vi "Main.vi"() -> ()   [LabVIEW 2017]
doc: "簡易ステートマシンデザインパターンを作成するのに、このテンプレートを使用します。各ステートはコードを実行して移行先のステートを決定します。"
uses:
  controls/State.ctl
  controls/Data.ctl
  controls/UI References.ctl
  controls/Graph Data.ctl
  controls/SQUID_data.ctl
  controls/XYZ_Data.ctl
  controls/HW Configuration.ctl
  controls/SQUID_configuration.ctl
  controls/SQUID_filter.ctl
  controls/SampleHandler_configuration.ctl
  controls/Degausser_configuration.ctl
  controls/Sequence_controll.ctl
  controls/Curret_status.ctl
  controls/wait_mode.ctl
  <vilib>/Utility/file.llb/Write Delimited Spreadsheet (string).vi
panel:
  in  "Home":bool
  out "実行中":bool
  in  "Pause":bool
  in  "Execute":bool
  in  "Save":bool
  in  "Sequence":bool
  in  "Connect":bool
  in  "Hardware setting":bool
  in  "Quit":bool
  out "文字列 2":string
  out "文字列":string
  out "RU":bool
  out "RD":bool
  out "Axis":string
  out "AF peak":u16
  out "Zero":bool
  out "Tracking":bool
  out "position (cm)":dbl
  out "Motor count":i32
  out "ARM":bool
  out "Degausser":bool
  out "Sample Handler":bool
  out "SQUID":bool
  out "数値":dbl
  out "Sequence":i32(listbox)
  out "command":i32(listbox)
  # "Status"
  # "Connection"
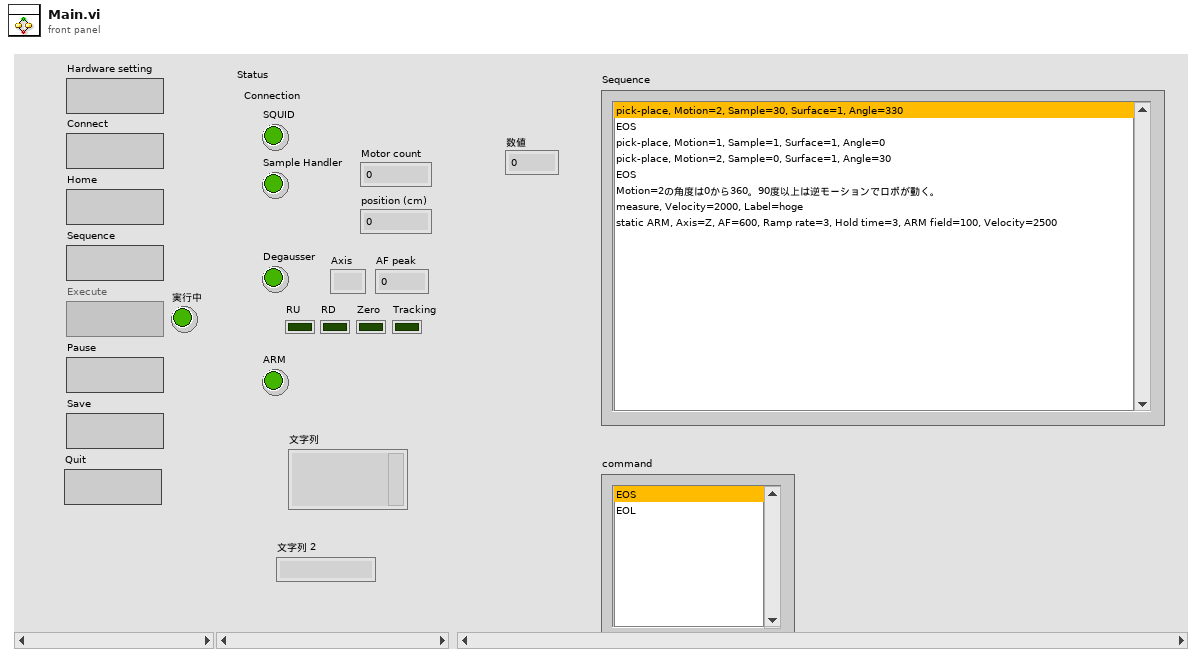
[diagram p1: front panel]
types:
  T1 = typedef "Data.ctl" = cluster{"UI ref":T2, "data":T3, "User":cluster{"Hardware configuration":T6}, "シーケンス制御":T11, "Current status":T12, "Sample offset":u16[]}
  T2 = typedef "UI References.ctl" = cluster{"Hardware setting":refnum<vi>, "Execute":refnum<vi>, "Sequence":refnum<vi>, "Pause":refnum<vi>, "Save":refnum<vi>, "Quit":refnum<vi>, "Connect":refnum<vi>}
  T3 = typedef "Graph Data.ctl" = cluster{"Label":string[], "Background":T4[], "Sample":T4[]}
  T4 = typedef "SQUID_data.ctl" = cluster{"reading":T5, "count":T5, "magnetization":T5}
  T5 = typedef "XYZ_Data.ctl" = cluster{"X":dbl, "Y":dbl, "Z":dbl}
  T6 = typedef "HW Configuration.ctl" = cluster{"SQUID":T7, "Sample Handler":T9, "Degausser":T10, "ARM Unit":cluster{"port":refnum<visa-resource-name>}, "IRM Unit（未実装）":cluster{"port":refnum<visa-resource-name>}, "Robot":cluster{"port":refnum<visa-resource-name>}}
  T7 = typedef "SQUID_configuration.ctl" = cluster{"port":refnum<visa-resource-name>, "Flux constant":T5, "X":T8, "Y":T8, "Z":T8}
  T8 = typedef "SQUID_filter.ctl" = u16
  T9 = typedef "SampleHandler_configuration.ctl" = cluster{"port":refnum<visa-resource-name>, "BG 1":i32, "BG 2":i32, "Sensor":i32, "AF 1":i32, "AF 2":i32, "AF coil":i32, "Home (absolute)":i32, "Home (relative to limit switch)":i32, "robot":i32}
  T10 = typedef "Degausser_configuration.ctl" = cluster{"port":refnum<visa-resource-name>, "Tracking timeout (sec)":i16, "Communication Delays":i16}
  T11 = typedef "Sequence_controll.ctl" = cluster{"実行中のシーケンス番号":u16, "実行中のコマンド番号":u16, "シーケンス配列":string[], "コマンド配列":string[]}
  T12 = typedef "Curret_status.ctl" = cluster{"Motor count":i32, "Degausser status":string, "Degausser axis":string, "wait mode":T13}
  T13 = typedef "wait_mode.ctl" = enum16{"Idle", "Executing", "Moving", "Homing", "Zeroing", "Ramping", "Robot", "Pause"}
  T14 = typedef "State.ctl" = enum16{"Initialize", "Update UI", "Wait for Event", "Hardware setting", "Connect", "Wait while executing", "Wait moving", "Wait homing", "Wait zero", "Wait tracking", "Wait robot", "Update command", "Exit", "Error"}
  T15 = typedef "HW_selection.ctl" = enum16{"Sample Handler", "SQUID", "Degausser", "ARM", "IRM", "Robot", "System", "Unknown"}
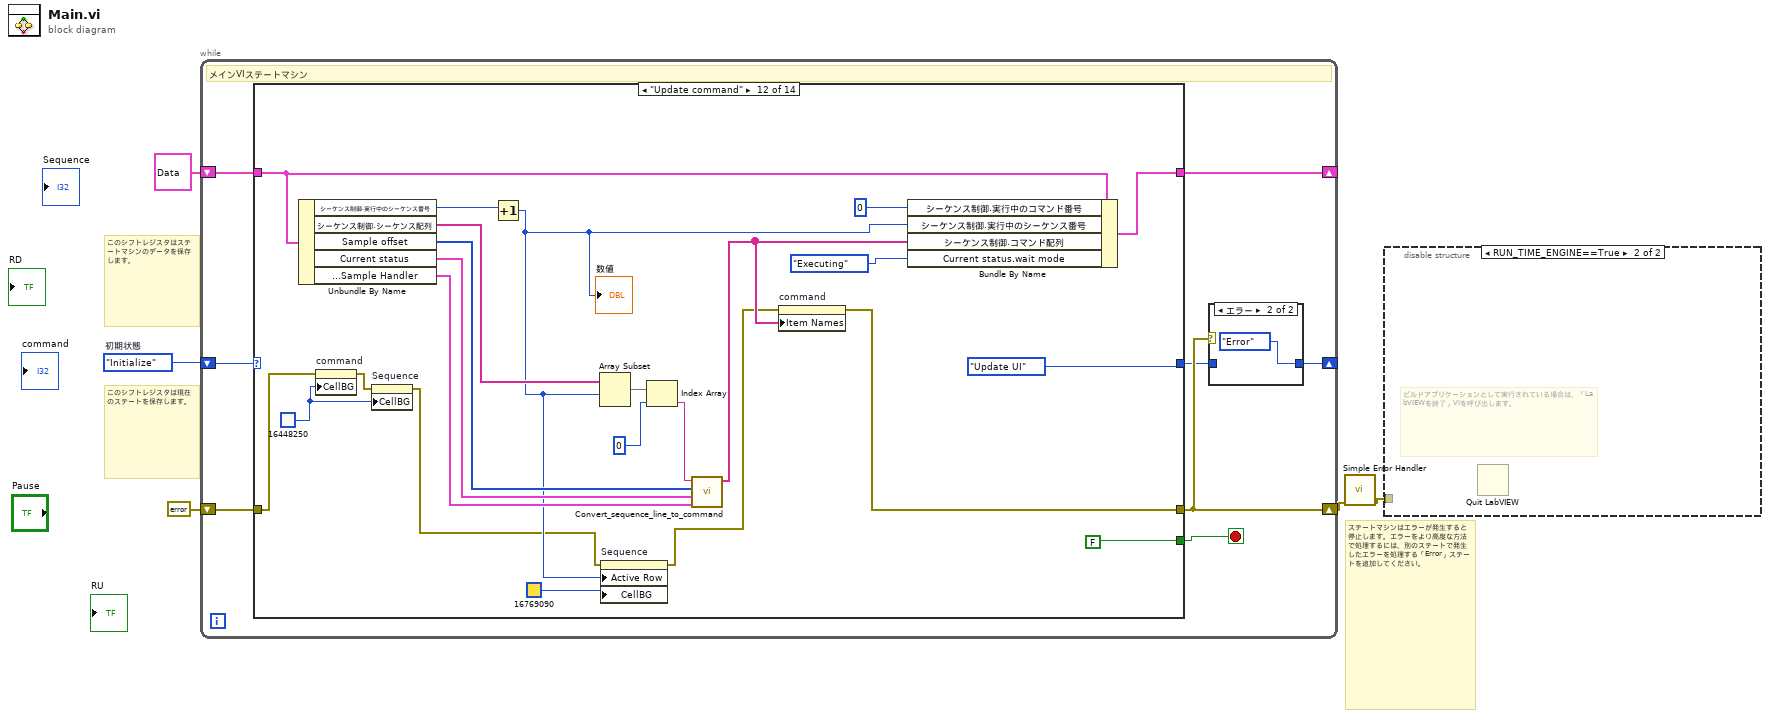
[diagram p0: block diagram]
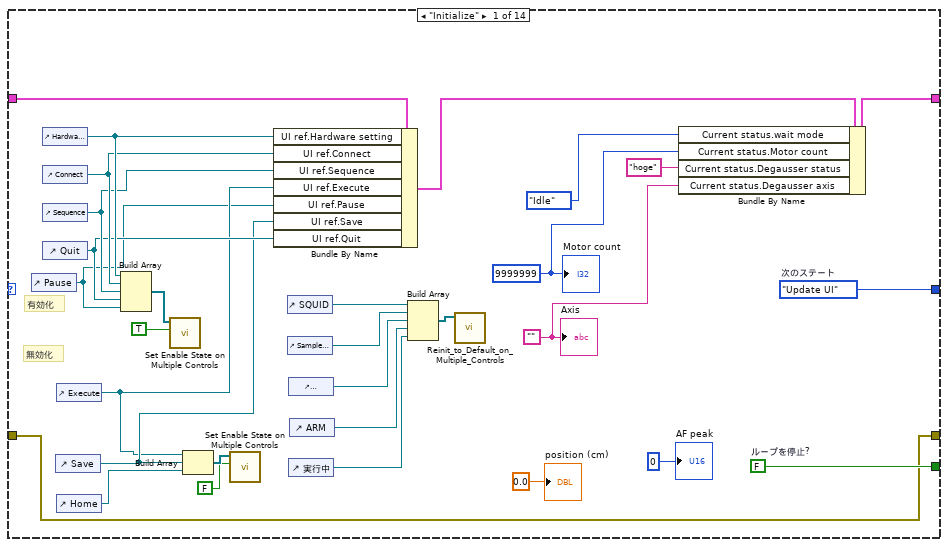
[diagram p4: hidden frame]
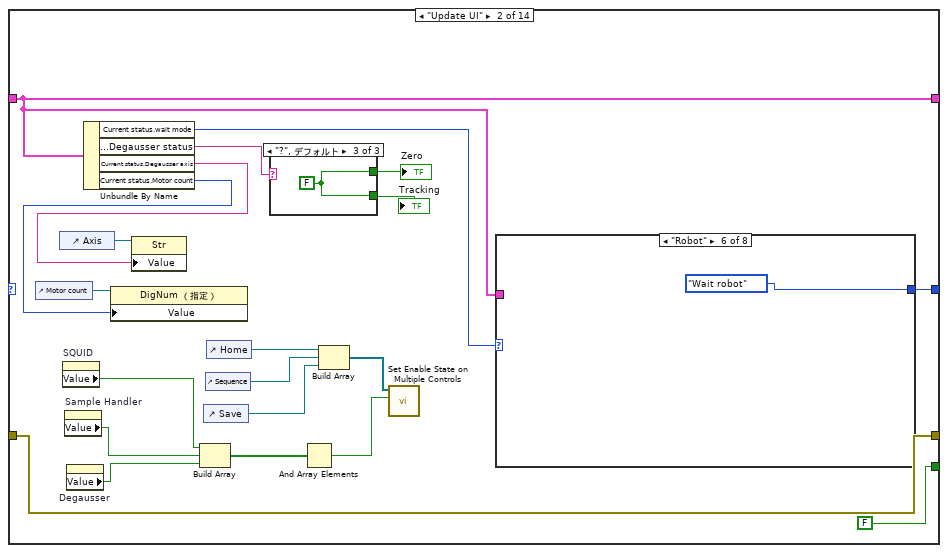
[diagram p5: hidden frame]
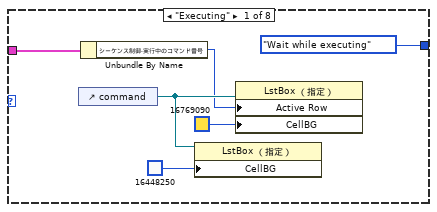
[diagram p6: hidden frame]
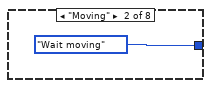
[diagram p7: hidden frame]
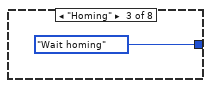
[diagram p8: hidden frame]
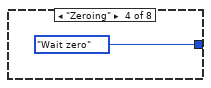
[diagram p9: hidden frame]
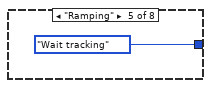
[diagram p10: hidden frame]
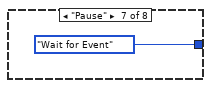
[diagram p11: hidden frame]
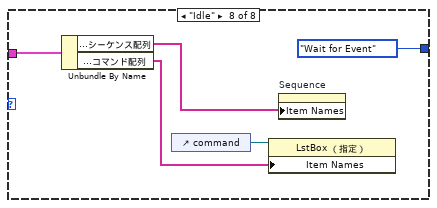
[diagram p12: hidden frame]
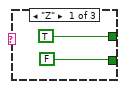
[diagram p13: hidden frame]
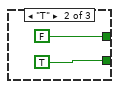
[diagram p14: hidden frame]
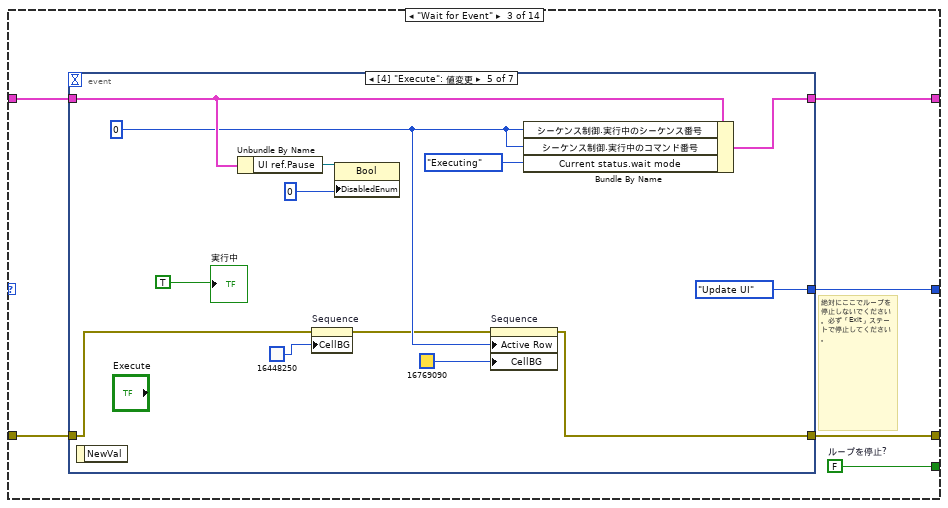
[diagram p15: hidden frame]
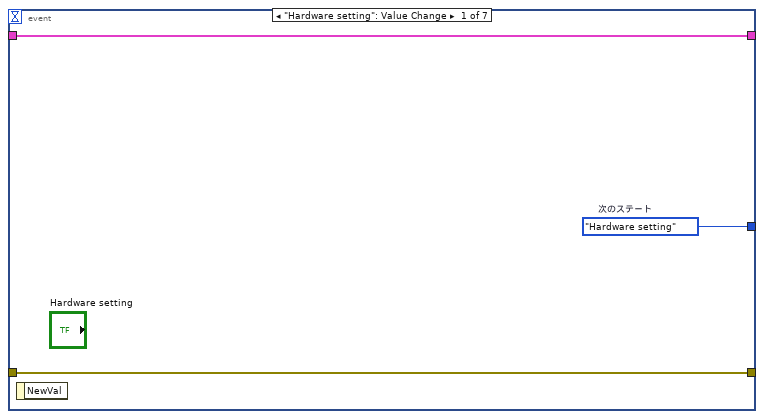
[diagram p16: hidden frame]
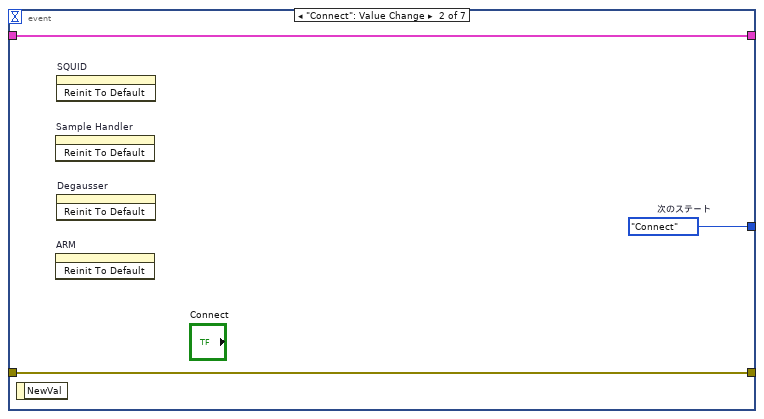
[diagram p17: hidden frame]
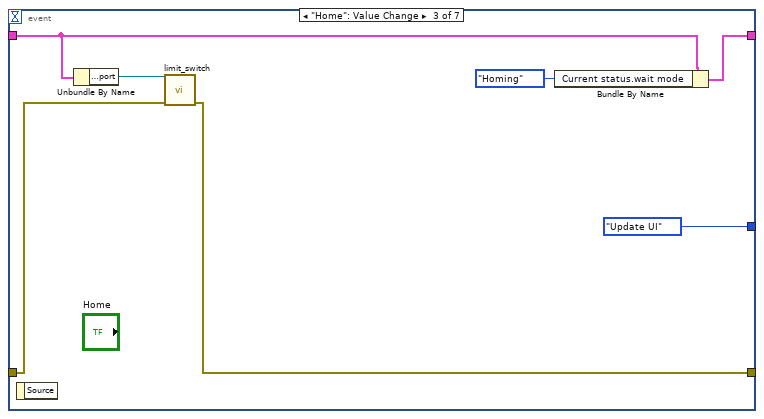
[diagram p18: hidden frame]
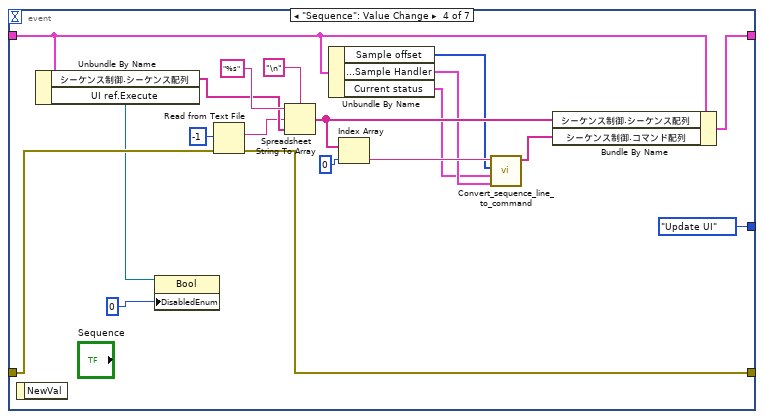
[diagram p19: hidden frame]
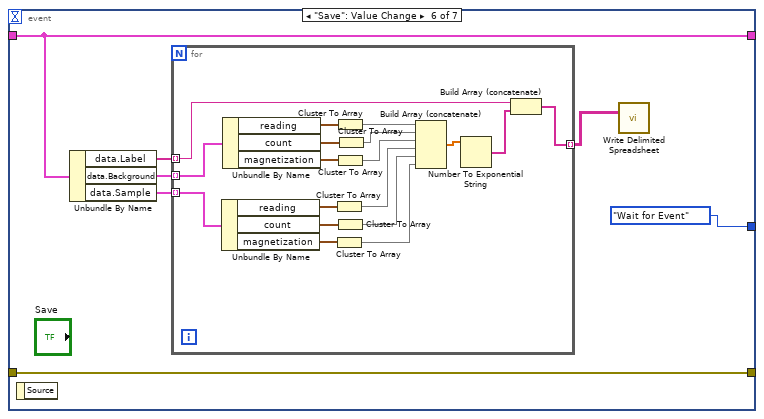
[diagram p20: hidden frame]
diagram:
  w5 = State."Initialize"  # 初期状態
  # "ステートマシンはエラーが発生すると停止します。エラーをより高度な方法で処理するには、別のステートで発生したエラーを処理する「Error」ステートを追加してください。"
  # "このシフトレジスタはステートマシンのデータを保存します。"
  # "このシフトレジスタは現在のステートを保存します。"
  n1 = while {
    shift-right: [w7] -> _
    shift-left: w5 -> [w13]
    shift-right: [w12] -> _
    shift-left: T1 {"UI ref"={"Hardware setting"=refnum, "Execute"=refnum, "Sequence"=refnum, "Pause"=refnum, "Save"=refnum, "Quit"=refnum, "Connect"=refnum}, "data"={"Label"=[], "Background"=[], "Sample"=[]}, "User"={"Hardware configuration"={"SQUID"={"port"="", "Flux constant"={"X"=0.0, "Y"=0.0, "Z"=0.0}, "X"=0, "Y"=0, "Z"=0}, "Sample Handler"={"port"="", "BG 1"=0, "BG 2"=0, "Sensor"=0, "AF 1"=0, "AF 2"=0, "AF coil"=0, "Home (absolute)"=0, "Home (relative to limit switch)"=0, "robot"=40750}, "Degausser"={"port"="", "Tracking timeout (sec)"=0, "Communication Delays"=0}, "ARM Unit"={"port"=""}, "IRM Unit（未実装）"={"port"=""}, "Robot"={"port"=""}}}, "シーケンス制御"={"実行中のシーケンス番号"=0, "実行中のコマンド番号"=0, "シーケンス配列"=[], "コマンド配列"=[]}, "Current status"={"Motor count"=0, "Degausser status"="", "Degausser axis"="", "wait mode"=enum."Idle"}, "Sample offset"=[37618]} ("Data") -> [w10]
    shift-right: [w9] -> w2
    shift-left: errorcluster {"status"=FALSE, "code"=0, "source"=""} ("error constant") -> [w11]
    stop <- w6 stop-if-true
    # "メインVIステートマシン"
    n2 = case shown="\"Update command\"" w13 {
      tunnel: [w45 w66 w94 w173 w199 w208 w406 w453 w492 w516 State."Wait tracking" ("ステート") State."Update UI" ("ステート") w588 State."Exit" ("ステート")] -> w8
      tunnel: [w44 FALSE w93 FALSE ("Stop Loop?") FALSE ("Stop Loop?") w214 FALSE FALSE FALSE FALSE FALSE FALSE w587 FALSE] -> w6
      tunnel: w10 -> [w34 w47 w92 w169 w197 w213 w403 w450 w495 w519 w545 w553 w578 w592]
      tunnel: [w23 w47 w91 w168 w196 w212 w402 w449 w494 w518 w545 w552 w578 w592] -> w12
      tunnel: w11 -> [w33 w56 w90 w171 w193 w211 w401 w448 w498 w521 w544 w563 w579 w591]
      tunnel: [w33 w56 w89 w171 w175 w209 w400 w447 w497 w515 w544 w557 w569 w591] -> w9
      frame "Initialize" {
        w19 = ""
        w21 = 9999999
        w44 = FALSE  # ループを停止?
        w45 = State."Update UI"  # 次のステート
        # "無効化"
        # "有効化"
        # "Initialize ― アプリケーションを初期化します。"
        n3 = control-ref of="Pause"() -> (w16:refnum<vi>)
        n4 = control-ref of="Hardware setting"() -> (w32:refnum<vi>)
        n5 = control-ref of="Connect"() -> (w31:refnum<vi>)
        n6 = control-ref of="Sequence"() -> (w30:refnum<vi>)
        n7 = control-ref of="Quit"() -> (w29:refnum<vi>)
        n8 = control-ref of="Save"() -> (w28:refnum<vi>)
        n9 = control-ref of="Execute"() -> (w17:refnum<vi>)
        n10 = control-ref of="Home"() -> (w18:refnum<vi>)
        n11 = Build Array(w32, w31, w30, w29, w16) -> (w43:refnum<vi>[])
        n12 = call "Set Enable State on Multiple Controls.vi"("有効?"=TRUE, "制御器"=w43) -> ()  [unwired: 10 in]
        n13 = Build Array(w17, w28, w18) -> (w41:refnum<vi>[])
        n14 = call "Set Enable State on Multiple Controls.vi"("有効?"=FALSE, "制御器"=w41) -> ()  [unwired: 10 in]
        n15 = Bundle By Name(cluster=w34, "UI ref.Hardware setting"=w32, "UI ref.Connect"=w31, "UI ref.Sequence"=w30, "UI ref.Execute"=w17, "UI ref.Pause"=w16, "UI ref.Save"=w28, "UI ref.Quit"=w29) -> (w24:T1)
        n16 = control-ref of="SQUID"() -> (w39:refnum<vi>)
        n17 = control-ref of="Sample Handler"() -> (w38:refnum<vi>)
        n18 = control-ref of="Degausser"() -> (w36:refnum<vi>)
        n19 = control-ref of="実行中"() -> (w22:refnum<vi>)
        n20 = control-ref of="ARM"() -> (w35:refnum<vi>)
        n21 = Build Array(w39, w38, w36, w35, w22) -> (w37:refnum<vi>[])
        n22 = call "Reinit_to_Default_on_Multiple_Controls.vi"("配列"=w37) -> ()  [unwired: 11 in]
        n23 = Bundle By Name(cluster=w24, "Current status.wait mode"=wait_mode."Idle" ("wait mode"), "Current status.Motor count"=w21, "Current status.Degausser status"="hoge", "Current status.Degausser axis"=w19) -> (w23:T1)
        "Motor count" <- w21
        "Axis" <- w19
        "AF peak" <- 0
        "position (cm)" <- 0.0
      }
      frame "Update UI" {
        n24 = control-ref of="Motor count"() -> (w60:refnum<vi>)
        n25 = control-ref of="Axis"() -> (w62:refnum<vi>)
        n26 = property on="SQUID" class="Bool （指定）"() -> ("Value"=w51:bool)  [unwired: 2 in, 2 out]
        n27 = property on="Sample Handler" class="Bool （指定）"() -> ("Value"=w50:bool)  [unwired: 2 in, 2 out]
        n28 = property on="Degausser" class="Bool （指定）"() -> ("Value"=w49:bool)  [unwired: 2 in, 2 out]
        n29 = Unbundle By Name(w47) -> ("Current status.wait mode"=w57:T13, "Current status.Degausser status"=w65:string, "Current status.Degausser axis"=w61:string, "Current status.Motor count"=w59:i32)
        n30 = property class="DigNum （指定）"(reference=w60, "Value"=w59) -> ()  [unwired: 1 in, 2 out]
        n31 = property class="Str"(reference=w62, "Value"=w61) -> ()  [unwired: 1 in, 2 out]
        n32 = Build Array(w51, w50, w49) -> (w48:bool[])
        n33 = control-ref of="Save"() -> (w46:refnum<vi>)
        n34 = control-ref of="Sequence"() -> (w52:refnum<vi>)
        n35 = control-ref of="Home"() -> (w53:refnum<vi>)
        n36 = case shown="\"?\", デフォルト" w65 {
          tunnel: [TRUE FALSE w88] -> w64
          tunnel: [FALSE TRUE w88] -> w63
          frame "Z" {
          }
          frame "T" {
          }
          frame "?", Default {
            w88 = FALSE
          }
        }
        "Zero" <- w64
        "Tracking" <- w63
        n37 = And Array Elements(Boolean array=w48) -> (logical AND=w54:bool)
        n38 = Build Array(w53, w52, w46) -> (w55:refnum<vi>[])
        n39 = call "Set Enable State on Multiple Controls.vi"("有効?"=w54, "制御器"=w55) -> ()  [unwired: 10 in]
        n40 = case shown="\"Robot\"" w57 {
          tunnel: [State."Wait while executing" ("ステート") State."Wait moving" ("ステート") State."Wait homing" ("ステート") State."Wait zero" ("ステート") State."Wait tracking" ("ステート") State."Wait robot" ("ステート") State."Wait for Event" ("ステート") State."Wait for Event" ("ステート")] -> w66
          tunnel: w47 -> [w68 _ _ _ _ _ _ w81]
          frame "Executing" {
            n41 = control-ref of="command"() -> (w71:refnum<vi>)
            n42 = Unbundle By Name(w68) -> ("シーケンス制御.実行中のコマンド番号"=w67:u16)
            n43 = property class="LstBox （指定）"(reference=w71, "CellBG"=u32 16448250) -> ()  [unwired: 1 in, 2 out]
            n44 = property class="LstBox （指定）"(reference=w71, "Active Row"=w67, "CellBG"=u32 16769090) -> ()  [unwired: 1 in, 2 out]
          }
          frame "Moving" {
          }
          frame "Homing" {
          }
          frame "Zeroing" {
          }
          frame "Ramping" {
          }
          frame "Robot" {
          }
          frame "Pause" {
          }
          frame "Idle" {
            n45 = Unbundle By Name(w81) -> ("シーケンス制御.シーケンス配列"=w79:string[], "シーケンス制御.コマンド配列"=w80:string[])
            n46 = control-ref of="command"() -> (w82:refnum<vi>)
            n47 = property class="LstBox （指定）"(reference=w82, "Item Names"=w80) -> ()  [unwired: 1 in, 2 out]
            n48 = property on="Sequence" class="LstBox （指定）"("Item Names"=w79) -> ()  [unwired: 2 in, 2 out]
          }
        }
      }
      frame "Wait for Event" {
        w93 = FALSE  # ループを停止?
        # "絶対にここでループを停止しないでください。必ず「Exit」ステートで停止してください。"
        # "Wait for Event - イベントストラクチャを使用し、ステートマシンの各ステートを実行するユーザインタフェースイベントの発生を監視します。"
        n49 = event shown="[4] \"Execute\": 値変更" {
          selector: _ -> [_ _ _ _ _ _ _]
          dyn-events: _ -> [_ _ _ _ _ _ _]
          timeout: _ -> [_ _ _ _ _ _ _]
          tunnel: [w97 w100 State."Update UI" ("ステート") State."Update UI" ("ステート") State."Update UI" ("ステート") State."Wait for Event" ("ステート") w167] -> w94
          tunnel: w92 -> [w95 w98 w105 w113 w136 w145 w166]
          tunnel: [w95 w98 w106 w123 w138 w145 w166] -> w91
          tunnel: w90 -> [w96 w99 w103 w126 w130 w146 w165]
          tunnel: [w96 w99 w102 w121 w127 w146 w165] -> w89
          event "Hardware setting": Value Change {
            w97 = State."Hardware setting"  # 次のステート
            n50 = event-data() -> ()  [unwired: 1 in, 1 out]
          }
          event "Connect": Value Change {
            w100 = State."Connect"  # 次のステート
            n51 = event-data() -> ()  [unwired: 1 in, 1 out]
            n52 = invoke on="Sample Handler" class="Bool （指定）" method="Reinit To Default"() -> ()  [unwired: 3 in, 3 out]
            n53 = invoke on="ARM" class="Bool （指定）" method="Reinit To Default"() -> ()  [unwired: 3 in, 3 out]
            n54 = invoke on="SQUID" class="Bool （指定）" method="Reinit To Default"() -> ()  [unwired: 3 in, 3 out]
            n55 = invoke on="Degausser" class="Bool （指定）" method="Reinit To Default"() -> ()  [unwired: 3 in, 3 out]
          }
          event "Home": Value Change {
            n56 = event-data() -> ()  [unwired: 1 in, 1 out]
            n57 = Unbundle By Name(w105) -> ("User.Hardware configuration.Sample Handler.port"=w104:refnum<visa-resource-name>)
            n58 = call "limit_switch.vi"("error in (no error)"=w103, "VISAリソース名"=w104) -> ("error out"=w102:errorcluster)  [unwired: 8 in, 1 out]
            n59 = Bundle By Name(cluster=w105, "Current status.wait mode"=wait_mode."Homing" ("wait mode")) -> (w106:T1)
          }
          event "Sequence": Value Change {
            n60 = event-data() -> ()  [unwired: 1 in, 1 out]
            n61 = Unbundle By Name(w113) -> ("シーケンス制御.シーケンス配列"=w109:string[], "UI ref.Execute"=w119:refnum<vi>)
            n62 = property class="Bool"(reference=w119, "DisabledEnum"=0) -> ()  [unwired: 1 in, 2 out]
            n63 = Read from Text File(count=-1, error in=w126) -> (text=w108:string, error out=w121:errorcluster)  [unwired: 2 in, 2 out]
            n64 = Spreadsheet String To Array(delimiter (Tab)="\n", format string="%s", spreadsheet string=w108, array type (2D Dbl)=w109) -> (array=w117:string[])
            n65 = Unbundle By Name(w113) -> ("Sample offset"=w110:u16[], "User.Hardware configuration.Sample Handler"=w112:T9, "Current status"=w111:T12)
            n66 = Index Array(array=w117, index=0) -> (element=w115:string)
            n67 = call "Convert_sequence_line_to_command.vi"("Sample Handler Configuration"=w112, "Current status"=w111, "Sample offset"=w110, "sequence line"=w115) -> ("コマンド配列"=w114:string[])  [unwired: 7 in]
            n68 = Bundle By Name(cluster=w113, "シーケンス制御.シーケンス配列"=w117, "シーケンス制御.コマンド配列"=w114) -> (w123:T1)
          }
          event "Execute": Value Change {
            w132 = 0
            n69 = event-data() -> ()  [unwired: 1 in, 1 out]
            n70 = Unbundle By Name(w136) -> ("UI ref.Pause"=w135:refnum<vi>)
            n71 = property on="Sequence" class="LstBox （指定）"(error in=w130, "CellBG"=u32 16448250) -> (error out=w128:errorcluster)  [unwired: 1 in, 1 out]
            n72 = property class="Bool"(reference=w135, "DisabledEnum"=0) -> ()  [unwired: 1 in, 2 out]
            n73 = property on="Sequence" class="LstBox （指定）"(error in=w128, "Active Row"=w132, "CellBG"=u32 16769090) -> (error out=w127:errorcluster)  [unwired: 1 in, 1 out]
            n74 = Bundle By Name(cluster=w136, "シーケンス制御.実行中のシーケンス番号"=w132, "シーケンス制御.実行中のコマンド番号"=w132, "Current status.wait mode"=wait_mode."Executing" ("wait mode")) -> (w138:T1)
            "実行中" <- TRUE
          }
          event "Save": Value Change {
            n75 = event-data() -> ()  [unwired: 1 in, 1 out]
            n76 = Unbundle By Name(w145) -> ("data.Label"=w140:string[], "data.Background"=w141:T4[], "data.Sample"=w144:T4[])
            n77 = for {
              tunnel: w144 -> [w160] mode=indexing
              tunnel: [w161] -> w143 mode=indexing
              tunnel: w141 -> [w156] mode=indexing
              tunnel: w140 -> [w148] mode=indexing
              n78 = Unbundle By Name(w160) -> ("reading"=w164:T5, "count"=w162:T5, "magnetization"=w163:T5)
              n79 = Unbundle By Name(w156) -> ("reading"=w159:T5, "count"=w157:T5, "magnetization"=w158:T5)
              n80 = Cluster To Array(cluster=w164) -> (array=w152:dbl[])
              n81 = Cluster To Array(cluster=w163) -> (array=w150:dbl[])
              n82 = Cluster To Array(cluster=w159) -> (array=w155:dbl[])
              n83 = Cluster To Array(cluster=w158) -> (array=w153:dbl[])
              n84 = Cluster To Array(cluster=w162) -> (array=w151:dbl[])
              n85 = Cluster To Array(cluster=w157) -> (array=w154:dbl[])
              n86 = Build Array (concatenate)(w155, w154, w153, w152, w151, w150) -> (w149:dbl[])
              n87 = Number To Exponential String(number=w149) -> (E-format string=w147:string[])  [unwired: 3 in]
              n88 = Build Array (concatenate)(w148, w147) -> (w161:string[])
            }
            n89 = call-poly <vilib>:"Write Delimited Spreadsheet.vi"("2D data"=w143) -> ()  [unwired: 13 in, 2 out]
          }
          event "Quit": Value Change {
            w167 = State."Exit"  # 次のステート
            n90 = event-data() -> ()  [unwired: 1 in, 1 out]
          }
        }
      }
      frame "Hardware setting" {
        w173 = State."Wait for Event"  # 次のステート
        # "User State 1 - このステートをユーザ自身のアプリケーションの機能と置換します。"
        n91 = call "Configure_HW_dialog.vi"() -> ("output"=w170:T6)  [unwired: 11 in]
        n92 = Bundle By Name(cluster=w169, "User.Hardware configuration"=w170) -> (w168:T1)
      }
      frame "Connect" {
        w199 = State."Update UI"  # 次のステート
        # "User State 2 - このステートをユーザ自身のアプリケーションの機能と置換します。"
        n93 = Unbundle By Name(w197) -> ("User.Hardware configuration.SQUID.port"=w194:refnum<visa-resource-name>, "User.Hardware configuration.Sample Handler.port"=w192:refnum<visa-resource-name>, "User.Hardware configuration.Degausser.port"=w189:refnum<visa-resource-name>, "User.Hardware configuration.Degausser.Communication Delays"=w188:i16, "User.Hardware configuration.ARM Unit.port"=w186:refnum<visa-resource-name>, "User.Hardware configuration.Robot.port"=w174:refnum<visa-resource-name>)
        n94 = call "test_connection_SQUID.vi"("error in (no error)"=w193, "VISAリソース名"=w194) -> ("error out"=w191:errorcluster, "connected?"=→"SQUID":bool, "VISAリソース名（出力）"=w185:refnum<visa-resource-name>)  [unwired: 7 in]
        n95 = call "test_connection_SampleHandler.vi"("error in (no error)"=w191, "VISAリソース名"=w192) -> ("error out"=w190:errorcluster, "Motor count"=w178:i32, "connected?"=→"Sample Handler":bool, "VISAリソース名（出力）"=w184:refnum<visa-resource-name>)  [unwired: 6 in]
        n96 = call "test_connection_Degausser.vi"("Character Delay"=w188, "error in (no error)"=w190, "VISAリソース名"=w189) -> ("error out"=w187:errorcluster, "connected?"=→"Degausser":bool, "VISAリソース名（出力）"=w183:refnum<visa-resource-name>)  [unwired: 6 in]
        n97 = call "test_connection_ARM.vi"("error in (no error)"=w187, "VISAリソース名"=w186) -> ("error out"=w177:errorcluster, "connected?"=→"ARM":bool, "VISAリソース名（出力）"=w182:refnum<visa-resource-name>)  [unwired: 7 in]
        n98 = flat-sequence {
          tunnel: w174 -> [w206]
          tunnel: w177 -> [w205]
          tunnel: [w201] -> w176
          tunnel: [w204] -> w175
          frame #0 {
            n99 = VISA Open(error in (no error)=w205, VISA resource name=w206) -> (VISA resource name=w202:refnum<visa-resource-name>, error out=w204:errorcluster)  [unwired: 3 in]
            n100 = property class="Instr"(reference=w202, "General Settings:Timeout Value"=u32 150000, "TermChar En"=TRUE) -> (reference out=w201:refnum<visa-resource-name>)  [unwired: 1 in, 1 out]
          }
          frame #1 {
            n101 = One Button Dialog(message="connect using robot PC") -> ()  [unwired: 1 in, 1 out]
          }
        }
        n102 = Bundle By Name(cluster=w197, "User.Hardware configuration.SQUID.port"=w185, "User.Hardware configuration.Sample Handler.port"=w184, "User.Hardware configuration.Degausser.port"=w183, "User.Hardware configuration.ARM Unit.port"=w182, "Current status.Motor count"=w178, "User.Hardware configuration.Robot.port"=w176) -> (w196:T1)
      }
      frame "Wait while executing" {
        n103 = event shown="[0] タイムアウト" {
          selector: _ -> [_ _]
          dyn-events: _ -> [_ _]
          timeout: 300 -> [_ _]
          tunnel: [FALSE FALSE] -> w214
          tunnel: w213 -> [w219 w398]
          tunnel: [w228 w398] -> w212
          tunnel: w211 -> [w225 w399]
          tunnel: [w215 State."Exit" ("ステート")] -> w208
          tunnel: [w221 w399] -> w209
          event Timeout {
            n104 = event-data() -> ()  [unwired: 1 in, 3 out]
            n105 = Unbundle By Name(w219) -> ("シーケンス制御.コマンド配列"=w229:string[], "シーケンス制御.実行中のコマンド番号"=w217:u16)
            n106 = Unbundle By Name(w219) -> ("UI ref.Execute"=w223:refnum<vi>)
            n107 = property class="Bool"(reference=w223, "DisabledEnum"=2) -> ()  [unwired: 1 in, 2 out]
            n108 = Index Array(array=w229, index=w217) -> (element=w216:string)
            n109 = call "categorize_command.vi"("command"=w216) -> ("HW"=w227:T15, "command (out)"=w226:string)  [unwired: 9 in]
            n110 = case shown="\"Robot\"" w227 {
              tunnel: w226 -> [w235 w284 w314 w322 w340 w372 _ _]
              tunnel: w219 -> [w241 w289 w316 w324 w343 w374 _ _]
              tunnel: w225 -> [w238 w287 w313 w321 w339 w371 w382 w392]
              tunnel: [w234 w286 w312 w320 w334 w368 w382 w392] -> w221
              tunnel: [wait_mode."Executing" ("wait mode") w285 wait_mode."Executing" ("wait mode") wait_mode."Executing" ("wait mode") wait_mode."Robot" ("wait mode") w367 w377 wait_mode."Executing" ("wait mode")] -> w220
              tunnel: w216 -> [w237 w283 _ _ _ w366 w378 _]
              tunnel: w219 -> [w232 w282 w311 w319 w331 w365 w380 w390]
              tunnel: [w231 w281 w311 w319 w330 w365 w380 w390] -> w218
              tunnel: [State."Update UI" ("ステート") State."Update UI" ("ステート") State."Update UI" ("ステート") State."Update UI" ("ステート") w332 State."Update UI" ("ステート") w379 State."Update UI" ("ステート")] -> w215
              frame "SQUID" {
                n111 = Unbundle By Name(w241) -> ("User.Hardware configuration.SQUID.port"=w236:refnum<visa-resource-name>, "User.Hardware configuration.SQUID.Flux constant"=w233:T5)
                n112 = case shown="\"measure\"" w237 {
                  selector: w237 -> [_ _ w265 _]
                  tunnel: w236 -> [w242 w261 _ w278]
                  tunnel: w238 -> [w246 w262 w266 w279]
                  tunnel: w235 -> [w247 _ _ _]
                  tunnel: [w244 w260 w266 w277] -> w234
                  tunnel: w233 -> [_ w255 _ w272]
                  tunnel: w232 -> [w243 w259 w270 w276]
                  tunnel: [w243 w254 w267 w271] -> w231
                  frame "ACLP" {
                    n113 = flat-sequence {
                      tunnel: w242 -> [w251]
                      tunnel: w247 -> [w250]
                      tunnel: w246 -> [w249]
                      tunnel: [w248] -> w245
                      tunnel: [w252] -> w244
                      tunnel: w245 -> [w252]
                      frame #0 {
                        n114 = call "one_by_one.vi"("error in (no error)"=w249, "入力文字"=w250, "VISAリソース名"=w251) -> ("error out"=w248:errorcluster)  [unwired: 7 in, 1 out]
                      }
                      frame #1 {
                        n115 = Wait (ms)(milliseconds to wait=1000) -> ()  [unwired: 1 out]
                      }
                    }
                  }
                  frame "measureBG" {
                    n116 = call "measure_once.vi"("error in (no error)"=w262, "flux constant"=w255, "VISAリソース名"=w261) -> ("error out"=w260:errorcluster, "SQUID data"=w257:T4)  [unwired: 6 in, 1 out]
                    n117 = Unbundle By Name(w259) -> ("data.Background"=w258:T4[])
                    n118 = Build Array (concatenate)(w258, w257) -> (w256:T4[])
                    n119 = Bundle By Name(cluster=w259, "data.Background"=w256) -> (w254:T1)
                  }
                  frame "label", Default {
                    n120 = Unbundle By Name(w270) -> ("data.Label"=w269:string[])
                    n121 = String Subset(string=w265, offset (0)=4) -> (substring=w263:string)  [unwired: 1 in]
                    n122 = Build Array (concatenate)(w269, w263) -> (w268:string[])
                    n123 = Bundle By Name(cluster=w270, "data.Label"=w268) -> (w267:T1)
                  }
                  frame "measure" {
                    n124 = call "measure_once.vi"("error in (no error)"=w279, "flux constant"=w272, "VISAリソース名"=w278) -> ("error out"=w277:errorcluster, "SQUID data"=w274:T4)  [unwired: 6 in, 1 out]
                    n125 = Unbundle By Name(w276) -> ("data.Sample"=w275:T4[])
                    n126 = Build Array (concatenate)(w275, w274) -> (w273:T4[])
                    n127 = Bundle By Name(cluster=w276, "data.Sample"=w273) -> (w271:T1)
                  }
                }
              }
              frame "Degausser" {
                n128 = Unbundle By Name(w289) -> ("User.Hardware configuration.Degausser.port"=w288:refnum<visa-resource-name>)
                n129 = call "one_by_one.vi"("error in (no error)"=w287, "入力文字"=w284, "VISAリソース名"=w288) -> ("error out"=w286:errorcluster)  [unwired: 7 in, 1 out]
                n130 = case shown="\"DERC\", \"DERD\"" w283 {
                  tunnel: [wait_mode."Executing" ("wait mode") wait_mode."Zeroing" ("wait mode") wait_mode."Executing" ("wait mode") wait_mode."Executing" ("wait mode") wait_mode."Executing" ("wait mode")] -> w285
                  tunnel: w282 -> [w290 w292 w296 w301 w306]
                  tunnel: [w290 w292 w294 w299 w304] -> w281
                  frame "else", Default {
                  }
                  frame "DERC", "DERD" {
                  }
                  frame "DCCX" {
                    n131 = Bundle By Name(cluster=w296, "Current status.Degausser axis"="X") -> (w294:T1)
                    n132 = Wait (ms)(milliseconds to wait=3000) -> ()  [unwired: 1 out]
                  }
                  frame "DCCY" {
                    n133 = Bundle By Name(cluster=w301, "Current status.Degausser axis"="Y") -> (w299:T1)
                    n134 = Wait (ms)(milliseconds to wait=3000) -> ()  [unwired: 1 out]
                  }
                  frame "DCCZ" {
                    n135 = Bundle By Name(cluster=w306, "Current status.Degausser axis"="Z") -> (w304:T1)
                    n136 = Wait (ms)(milliseconds to wait=3000) -> ()  [unwired: 1 out]
                  }
                }
              }
              frame "ARM" {
                n137 = Unbundle By Name(w316) -> ("User.Hardware configuration.ARM Unit.port"=w315:refnum<visa-resource-name>)
                n138 = call "one_by_one.vi"("error in (no error)"=w313, "入力文字"=w314, "VISAリソース名"=w315) -> ("error out"=w312:errorcluster)  [unwired: 7 in, 1 out]
              }
              frame "IRM" {
                n139 = Unbundle By Name(w324) -> ("User.Hardware configuration.IRM Unit（未実装）.port"=w323:refnum<visa-resource-name>)
                n140 = call "one_by_one.vi"("error in (no error)"=w321, "入力文字"=w322, "VISAリソース名"=w323) -> ("error out"=w320:errorcluster)  [unwired: 7 in, 1 out]
              }
              frame "Robot" {
                n141 = Unbundle By Name(w343) -> ("User.Hardware configuration.Robot.port"=w341:refnum<visa-resource-name>)
                n142 = flat-sequence {
                  tunnel: w341 -> [w350]
                  tunnel: w340 -> [w349]
                  tunnel: w339 -> [w348]
                  tunnel: [w347] -> w337
                  tunnel: [w346] -> w335
                  tunnel: [w352] -> w338
                  tunnel: w337 -> [w352]
                  tunnel: [w351] -> w336
                  tunnel: w335 -> [w351]
                  tunnel: w338 -> [w358]
                  tunnel: w336 -> [w359]
                  tunnel: [w356] -> w328
                  tunnel: [w355] -> w327
                  tunnel: [w354] -> w326
                  tunnel: [w362] -> w329
                  tunnel: [w363] -> w334
                  tunnel: w328 -> [w363]
                  tunnel: w327 -> [w362]
                  tunnel: w326 -> [w360]
                  tunnel: [w360] -> w325
                  frame #0 {
                    n143 = VISA Write(VISA resource name=w350, write buffer=w349, error in (no error)=w348) -> (VISA resource name out=w347:refnum<visa-resource-name>, error out=w346:errorcluster)  [unwired: 1 out]
                  }
                  frame #1 {
                    n144 = Wait (ms)(milliseconds to wait=100) -> ()  [unwired: 1 out]
                  }
                  frame #2 {
                    n145 = VISA Read(VISA resource name=w358, byte count=6, error in (no error)=w359) -> (VISA resource name out=w354:refnum<visa-resource-name>, read buffer=w355:string, error out=w356:errorcluster)  [unwired: 1 out]
                  }
                  frame #3 {
                    n146 = Wait (ms)(milliseconds to wait=100) -> ()  [unwired: 1 out]
                  }
                }
                n147 = Bundle By Name(cluster=w331, "User.Hardware configuration.Robot.port"=w325) -> (w330:T1)
                n148 = call <vilib>:"Trim Whitespace.vi"("string"=w329) -> ("trimmed string"=w333:string)  [unwired: 1 in]
                n149 = case shown="\"10\"" w333 {
                  tunnel: [State."Error" ("ステート") State."Update UI" ("ステート")] -> w332
                  frame "FALSE", Default {
                  }
                  frame "10" {
                  }
                }
                "文字列 2" <- w329
              }
              frame "Sample Handler" {
                n150 = Unbundle By Name(w374) -> ("User.Hardware configuration.Sample Handler.port"=w373:refnum<visa-resource-name>)
                n151 = call "one_by_one.vi"("error in (no error)"=w371, "入力文字"=w372, "VISAリソース名"=w373) -> ("error out"=w369:errorcluster, "VISAリソース名出力"=w370:refnum<visa-resource-name>)  [unwired: 7 in]
                n152 = call "get_SampleHandler_state.vi"("error in (no error)"=w369, "VISAリソース名"=w370) -> ("error out"=w368:errorcluster)  [unwired: 7 in, 2 out]
                n153 = case shown="\"else\", デフォルト" w366 {
                  tunnel: [wait_mode."Executing" ("wait mode") wait_mode."Moving" ("wait mode")] -> w367
                  frame "else", Default {
                  }
                  frame "G" {
                  }
                }
              }
              frame "System" {
                n154 = Wait (ms)(milliseconds to wait=1000) -> ()  [unwired: 1 out]
                n155 = case shown="\"EOS\"" w378 {
                  tunnel: [State."Update UI" ("ステート") State."Update command" ("ステート") State."Update UI" ("ステート")] -> w379
                  tunnel: [wait_mode."Executing" ("wait mode") wait_mode."Executing" ("wait mode") wait_mode."Idle" ("wait mode")] -> w377
                  frame "else", Default {
                  }
                  frame "EOL" {
                  }
                  frame "EOS" {
                    n156 = invoke on="実行中" class="Bool （指定）" method="Reinit To Default"() -> ()  [unwired: 3 in, 3 out]
                  }
                }
              }
              frame "Unknown", Default {
              }
            }
            n157 = Increment(x=w217) -> (x+1=w224:u16)
            n158 = Bundle By Name(cluster=w218, "シーケンス制御.実行中のコマンド番号"=w224, "Current status.wait mode"=w220) -> (w228:T1)
          }
          event "Pause": Value Change {
            n159 = event-data() -> ()  [unwired: 1 in, 6 out]
            n160 = control-ref of="Pause"() -> (w395:refnum<vi>)
            n161 = property class="Bool" props=["Value"](reference=w395) -> (reference out=w394:refnum<vi>, error out=w393:errorcluster)  [unwired: 1 in, 1 out]
            n162 = invoke class="Bool" method="Reinit To Default"(reference=w394, error in=w393) -> ()  [unwired: 1 in, 3 out]
          }
        }
      }
      frame "Wait moving" {
        n163 = event shown="[1] \"Pause\": 値変更" {
          selector: _ -> [_ _]
          dyn-events: _ -> [_ _]
          timeout: 200 -> [_ _]
          tunnel: [w415 State."Exit" ("ステート")] -> w406
          tunnel: w403 -> [w413 w443]
          tunnel: [w414 w442] -> w402
          tunnel: w401 -> [w407 w445]
          tunnel: [w412 w445] -> w400
          event Timeout {
            n164 = event-data() -> ()  [unwired: 1 in, 1 out]
            n165 = Unbundle By Name(w413) -> ("User.Hardware configuration.Sample Handler.port"=w408:refnum<visa-resource-name>)
            n166 = call "get_SampleHandler_state.vi"("error in (no error)"=w407, "VISAリソース名"=w408) -> ("error out"=w409:errorcluster, "response"=w410:string, "VISAリソース名（出力）"=w411:refnum<visa-resource-name>)  [unwired: 7 in]
            n167 = case shown="\"5\"" w410 {
              tunnel: [State."Update UI" ("ステート") State."Wait moving" ("ステート") State."Wait moving" ("ステート")] -> w415
              tunnel: [w427 w437 w439] -> w414
              tunnel: w411 -> [w424 _ _]
              tunnel: w409 -> [w423 w436 w440]
              tunnel: w413 -> [w428 w437 w439]
              tunnel: [w420 w436 w440] -> w412
              frame "5" {
                # "なぜ二回必要なのか謎"
                n168 = call "VP.vi"("error in (no error)"=w423, "VISAリソース名"=w424) -> ("error out"=w422:errorcluster, "VISAリソース名（出力）"=w421:refnum<visa-resource-name>)  [unwired: 7 in, 1 out]
                n169 = call "VP.vi"("error in (no error)"=w422, "VISAリソース名"=w421) -> ("error out"=w420:errorcluster, "Motor count"=w418:i32)  [unwired: 7 in, 1 out]
                n170 = Bundle By Name(cluster=w428, "Current status.Motor count"=w418) -> (w417:T1)
                n171 = Unbundle By Name(w417) -> ("Current status.wait mode"=w419:T13)
                n172 = property on="実行中" class="Bool （指定）"() -> ("Value"=w426:bool)  [unwired: 2 in, 2 out]
                n173 = case shown="\"Idle\", デフォルト" w419 {
                  tunnel: w417 -> [w430 w433]
                  tunnel: w418 -> [_ w432]
                  tunnel: [w430 w431] -> w416
                  frame "Idle", Default {
                  }
                  frame "Homing" {
                    n174 = Bundle By Name(cluster=w433, "User.Hardware configuration.Sample Handler.Home (absolute)"=w432) -> (w431:T1)
                  }
                }
                n175 = case shown="FALSE" w426 {
                  tunnel: [wait_mode."Idle" ("wait mode") wait_mode."Executing" ("wait mode")] -> w425
                  frame False {
                  }
                  frame True {
                  }
                }
                n176 = Bundle By Name(cluster=w416, "Current status.wait mode"=w425) -> (w427:T1)
              }
              frame "7" {
              }
              frame "0", "G", Default {
              }
            }
          }
          event "Pause": Value Change {
            n177 = event-data() -> ()  [unwired: 1 in, 6 out]
            n178 = invoke on="Execute" class="Bool" method="Reinit To Default"() -> ()  [unwired: 3 in, 3 out]
            n179 = invoke on="Pause" class="Bool" method="Reinit To Default"() -> ()  [unwired: 3 in, 3 out]
            n180 = Bundle By Name(cluster=w443, "Current status.wait mode"=wait_mode."Idle" ("wait mode")) -> (w442:T1)
          }
        }
      }
      frame "Wait homing" {
        n181 = event shown="[0] タイムアウト" {
          selector: _ -> [_ _]
          dyn-events: _ -> [_ _]
          timeout: 100 -> [_ _]
          tunnel: [w462 State."Wait for Event" ("ステート")] -> w453
          tunnel: w450 -> [w461 w487]
          tunnel: [w459 w487] -> w449
          tunnel: w448 -> [w458 w486]
          tunnel: [w460 w486] -> w447
          event Timeout {
            n182 = event-data() -> ()  [unwired: 1 in, 3 out]
            n183 = Unbundle By Name(w461) -> ("User.Hardware configuration.Sample Handler.port"=w456:refnum<visa-resource-name>)
            n184 = call "get_SampleHandler_state.vi"("error in (no error)"=w458, "VISAリソース名"=w456) -> ("error out"=w457:errorcluster, "response"=w454:string, "VISAリソース名（出力）"=w455:refnum<visa-resource-name>)  [unwired: 7 in]
            n185 = case shown="\"7\"" w454 {
              tunnel: [State."Wait moving" ("ステート") State."Wait homing" ("ステート")] -> w462
              tunnel: w455 -> [w465 _]
              tunnel: w461 -> [w469 w483]
              tunnel: w457 -> [w464 w484]
              tunnel: [w471 w484] -> w460
              tunnel: [w468 w483] -> w459
              frame "7" {
                # "ここで戻さないのがミソ"
                n186 = Bundle By Name(cluster=w469, "Current status.wait mode"=wait_mode."Homing" ("wait mode")) -> (w468:T1)
                n187 = flat-sequence {
                  tunnel: w464 -> [w476]
                  tunnel: w467 -> [w475]
                  tunnel: [w477] -> w466
                  tunnel: w465 -> [w474]
                  tunnel: [w473] -> w463
                  tunnel: [w482] -> w471
                  tunnel: w466 -> [w482]
                  tunnel: w463 -> [w480]
                  frame #0 {
                    n188 = call "G.vi"("error in (no error)"=w476, "distance"=w475, "direction (+/-)"="+", "VISAリソース名"=w474) -> ("error out"=w477:errorcluster, "VISAリソース名（出力）"=w473:refnum<visa-resource-name>)  [unwired: 6 in]
                  }
                  frame #1 {
                    n189 = Wait (ms)(milliseconds to wait=2000) -> ()  [unwired: 1 out]
                    n190 = VISA Write(VISA resource name=w480, write buffer="Z") -> ()  [unwired: 1 in, 3 out]
                  }
                }
                n191 = Unbundle By Name(w468) -> ("User.Hardware configuration.Sample Handler.Home (relative to limit switch)"=w467:i32)
              }
              frame "0", "G", Default {
              }
            }
          }
          event "Pause": Value Change {
            n192 = event-data() -> ()  [unwired: 1 in, 6 out]
            n193 = control-ref of="Execute"() -> (w489:refnum<vi>)
            n194 = property class="Bool" props=["Value"](reference=w489) -> (reference out=w491:refnum<vi>, error out=w490:errorcluster)  [unwired: 1 in, 1 out]
            n195 = invoke class="Bool" method="Reinit To Default"(reference=w491, error in=w490) -> ()  [unwired: 1 in, 3 out]
          }
        }
      }
      frame "Wait zero" {
        n196 = event shown="[1] \"Pause\": 値変更" {
          selector: _ -> [_ _]
          dyn-events: _ -> [_ _]
          timeout: 1000 -> [_ _]
          tunnel: w498 -> [w508 _]
          tunnel: [w507 _] -> w497
          tunnel: w495 -> [w506 w513]
          tunnel: [w505 w511] -> w494
          tunnel: [State."Update UI" ("ステート") State."Wait for Event" ("ステート")] -> w492
          event Timeout {
            n197 = event-data() -> ()  [unwired: 1 in, 3 out]
            n198 = Unbundle By Name(w506) -> ("User.Hardware configuration.Degausser.port"=w503:refnum<visa-resource-name>, "User.Hardware configuration.Degausser.Communication Delays"=w504:i16)
            n199 = call "DSS.vi"("VISAリソース名"=w503, "文字列待機 (350 ms)"=w504, "error in (no error)"=w508) -> ("Status"=w502:string, "error out"=w507:errorcluster)  [unwired: 6 in, 5 out]
            n200 = Bundle By Name(cluster=w506, "Current status.Degausser status"=w502) -> (w500:T1)
            n201 = case shown="\"Z\"" w502 {
              tunnel: [wait_mode."Zeroing" ("wait mode") wait_mode."Executing" ("wait mode")] -> w501
              frame "FALSE", Default {
              }
              frame "Z" {
              }
            }
            n202 = Bundle By Name(cluster=w500, "Current status.wait mode"=w501) -> (w505:T1)
          }
          event "Pause": Value Change {
            n203 = event-data() -> ()  [unwired: 1 in, 6 out]
            n204 = Bundle By Name(cluster=w513, "Current status.wait mode"=wait_mode."Pause" ("wait mode")) -> (w511:T1)
          }
        }
      }
      frame "Wait robot" {
        n205 = event shown="[0] タイムアウト" {
          selector: _ -> [_ _]
          dyn-events: _ -> [_ _]
          timeout: 200 -> [_ _]
          tunnel: w521 -> [w532 _]
          tunnel: w519 -> [w525 w540]
          tunnel: [w530 w538] -> w518
          tunnel: [w531 State."Exit" ("ステート")] -> w516
          tunnel: [w529 _] -> w515
          event Timeout {
            n206 = event-data() -> ()  [unwired: 1 in, 3 out]
            n207 = Unbundle By Name(w525) -> ("User.Hardware configuration.Robot.port"=w522:refnum<visa-resource-name>)
            n208 = VISA Read(VISA resource name=w522, byte count=6, error in (no error)=w532) -> (VISA resource name out=w526:refnum<visa-resource-name>, read buffer=w523:string, error out=w529:errorcluster)  [unwired: 1 out]
            "文字列" <- w523
            n209 = call <vilib>:"Trim Whitespace.vi"("string"=w523) -> ("trimmed string"=w528:string)  [unwired: 1 in]
            n210 = case shown="\"\", デフォルト" w528 {
              tunnel: [wait_mode."Idle" ("wait mode") wait_mode."Executing" ("wait mode")] -> w533
              tunnel: [State."Exit" ("ステート") State."Update UI" ("ステート")] -> w531
              frame "", Default {
              }
              frame "20" {
              }
            }
            n211 = Bundle By Name(cluster=w525, "User.Hardware configuration.Robot.port"=w526) -> (w524:T1)
            n212 = Bundle By Name(cluster=w524, "Current status.wait mode"=w533) -> (w530:T1)
          }
          event "Pause": Value Change {
            n213 = event-data() -> ()  [unwired: 1 in, 6 out]
            n214 = invoke on="実行中" class="Bool （指定）" method="Reinit To Default"() -> ()  [unwired: 3 in, 3 out]
            n215 = invoke on="Pause" class="Bool" method="Reinit To Default"() -> ()  [unwired: 3 in, 3 out]
            n216 = Bundle By Name(cluster=w540, "Current status.wait mode"=wait_mode."Pause" ("wait mode")) -> (w538:T1)
          }
        }
      }
      frame "Wait tracking" {
      }
      frame "Update command" {
        w549 = u32 16448250
        n217 = Unbundle By Name(w553) -> ("シーケンス制御.実行中のシーケンス番号"=w566:u16, "シーケンス制御.シーケンス配列"=w562:string[], "Sample offset"=w561:u16[], "Current status"=w560:T12, "User.Hardware configuration.Sample Handler"=w559:T9)
        n218 = property on="command" class="LstBox （指定）"(error in=w563, "CellBG"=w549) -> (error out=w548:errorcluster)  [unwired: 1 in, 1 out]
        n219 = property on="Sequence" class="LstBox （指定）"(error in=w548, "CellBG"=w549) -> (error out=w547:errorcluster)  [unwired: 1 in, 1 out]
        n220 = Increment(x=w566) -> (x+1=w550:u16)
        "数値" <- w550
        n221 = Array Subset(array=w562, index=w550) -> (w565:string[])  [unwired: 1 in]
        n222 = property on="Sequence" class="LstBox （指定）"(error in=w547, "Active Row"=w550, "CellBG"=u32 16769090) -> (error out=w546:errorcluster)  [unwired: 1 in, 1 out]
        n223 = Index Array(array=w565, index=0) -> (element=w554:string)
        n224 = call "Convert_sequence_line_to_command.vi"("Sample Handler Configuration"=w559, "Current status"=w560, "Sample offset"=w561, "sequence line"=w554) -> ("コマンド配列"=w558:string[])  [unwired: 7 in]
        n225 = property on="command" class="LstBox （指定）"(error in=w546, "Item Names"=w558) -> (error out=w557:errorcluster)  [unwired: 1 in, 1 out]
        n226 = Bundle By Name(cluster=w553, "シーケンス制御.実行中のコマンド番号"=0, "シーケンス制御.実行中のシーケンス番号"=w550, "シーケンス制御.コマンド配列"=w558, "Current status.wait mode"=wait_mode."Executing" ("wait mode")) -> (w552:T1)
      }
      frame "Exit" {
        w587 = TRUE  # ループを停止?
        w588 = State."Exit"  # （値未使用）
        # "これはステートマシンループの最後の反復であるため、ステート値はここでは使用されません。"
        # "Exit - アプリケーションを終了します。"
        n227 = Unbundle By Name(w578) -> ("User.Hardware configuration.SQUID.port"=w586:refnum<visa-resource-name>, "User.Hardware configuration.Sample Handler.port"=w585:refnum<visa-resource-name>, "User.Hardware configuration.Degausser.port"=w581:refnum<visa-resource-name>, "User.Hardware configuration.ARM Unit.port"=w580:refnum<visa-resource-name>, "User.Hardware configuration.Robot.port"=w570:refnum<visa-resource-name>)
        n228 = control-ref of="Sample Handler"() -> (w576:refnum<vi>)
        n229 = control-ref of="Degausser"() -> (w575:refnum<vi>)
        n230 = control-ref of="ARM"() -> (w574:refnum<vi>)
        n231 = control-ref of="実行中"() -> (w572:refnum<vi>)
        n232 = control-ref of="SQUID"() -> (w577:refnum<vi>)
        n233 = Build Array(w577, w576, w575, w574, w572) -> (w573:refnum<vi>[])
        n234 = call "Reinit_to_Default_on_Multiple_Controls.vi"("配列"=w573) -> ()  [unwired: 11 in]
        n235 = VISA Close(VISA resource name=w586, error in (no error)=w579) -> (error out=w584:errorcluster)
        n236 = VISA Close(VISA resource name=w585, error in (no error)=w584) -> (error out=w583:errorcluster)
        n237 = VISA Close(VISA resource name=w581, error in (no error)=w583) -> (error out=w582:errorcluster)
        n238 = VISA Close(VISA resource name=w580, error in (no error)=w582) -> (error out=w571:errorcluster)
        n239 = VISA Close(VISA resource name=w570, error in (no error)=w571) -> (error out=w569:errorcluster)
      }
      frame "Error" {
      }
    }
    n240 = case shown="エラー" w9 {
      tunnel: w8 -> [w14 _]
      tunnel: [w14 State."Error" ("ステート")] -> w7
      frame No Error {
      }
      frame Error {
      }
    }
  }
  n241 = call <vilib>:"Simple Error Handler.vi"("error in (no error)"=w2) -> ("error out"=w1:errorcluster)  [unwired: 4 in, 4 out]
  n242 = disable-structure shown="RUN_TIME_ENGINE==True" {
    disable-tunnel: w1 -> [_ _]
    frame condition #0 (active) {
    }
    frame condition #1 {
      # "ビルドアプリケーションとして実行されている場合は、「LabVIEWを終了」VIを呼び出します。"
      n243 = Quit LabVIEW() -> ()  [unwired: 1 in]
    }
  }
